vi "Write UI VI Ref.vi"(8 "error in (no error)":errorcluster, 10 "UI VI Ref":refnum<vi>, 11 "ViewableActorEncaps in":refnum<class "ViewableActorEncaps.lvclass">) -> (0 "error out":errorcluster, 3 "ViewableActorEncaps out":refnum<class "ViewableActorEncaps.lvclass">)   [LabVIEW 2014, in "ViewableActor.lvlib" / "ViewableActorEncaps.lvclass"]
uses:
  ViewableActorEncaps.lvclass
  ViewableActor/ViewableActor.lvclass/ViewableActor.ctl
  ViewableActor/Read UI VI Ref.vi
  ViewableActor/ViewableActor.lvclass
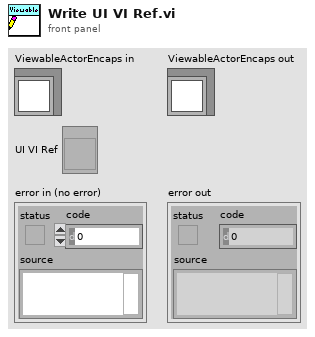
[diagram p1: front panel]
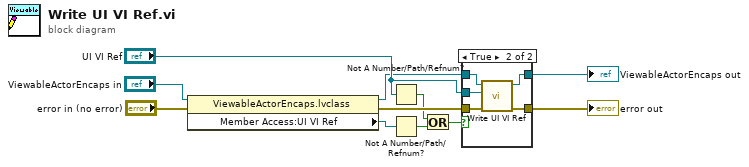
[diagram p0: block diagram]
diagram:
  n1 = property class="ViewableActorEncaps.lvclass"(reference="ViewableActorEncaps in", error in="error in (no error)") -> (reference out=w6:refnum<class "ViewableActorEncaps.lvclass">, error out=w5:errorcluster, "Member Access:UI VI Ref"=w4:refnum<vi>)
  n2 = Not A Number/Path/Refnum?(number/path/refnum="UI VI Ref") -> (NaN/Path/Refnum?=w1:bool)
  n3 = Not A Number/Path/Refnum?(number/path/refnum=w4) -> (NaN/Path/Refnum?=w3:bool)
  n4 = Or(x=w1, y=w3) -> (x .or. y?=w2:bool)
  n5 = case shown="True" w2 {
    tunnel: [w12 w18] -> w11
    tunnel: [w13 w17] -> w10
    tunnel: "UI VI Ref" -> [_ w16]
    tunnel: w6 -> [w13 w15]
    tunnel: w5 -> [w12 w14]
    frame False {
    }
    frame True {
      n6 = call-parent "Write UI VI Ref.vi"("error in (no error)"=w14, "UI VI Ref"=w16, "ViewableActor in"=w15) -> ("error out"=w18:errorcluster, "ViewableActor out"=w17:refnum<class "ViewableActorEncaps.lvclass">)  [unwired: 7 in]
    }
  }
  "error out" <- w11
  "ViewableActorEncaps out" <- w10
